vi "Legendre Polynomial.vi"(8 "type":i32(ring) items=["Standard", "Semi-Normalized", "Normalized"], 9 "m":i32, 10 "n":i32, 11 "x":dbl) -> (0 "error":i32, 3 "Legendre (n,m,x)":dbl)   [LabVIEW 2020, in "NI_AAL_Polynomial.lvlib"]
doc: "Calculates the associated Legendre polynomial of degree <B>n</B> and order <B>m</B> at point <B>x</B>."
uses:
  <vilib>/Analysis/NI_AAL_Polynomial.lvlib
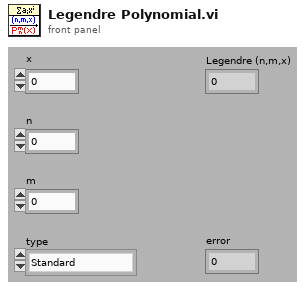
[diagram p1: front panel]
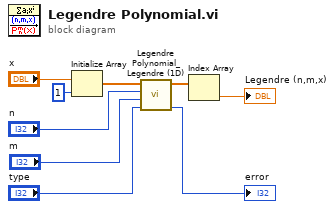
[diagram p0: block diagram]
diagram:
  n1 = Initialize Array("x", 1 ("dimension size")) -> (w7:dbl[])
  n2 = call <vilib>:"Legendre Polynomial_Legendre (1D).vi"("type"="type", "m"="m", "n"="n", "X"=w7) -> ("error"=→"error":i32, "Legendre (n,m,X)"=w3:dbl[])  [unwired: 6 in]
  n3 = Index Array(array=w3) -> (element=→"Legendre (n,m,x)":dbl)  [unwired: 1 in]
